vi "RNG.vi"(9 "Minim":dbl, 10 "Maxim":dbl) -> (2 "X val aleatoare":dbl)   [LabVIEW 2024]
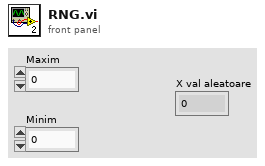
[diagram p1: front panel]
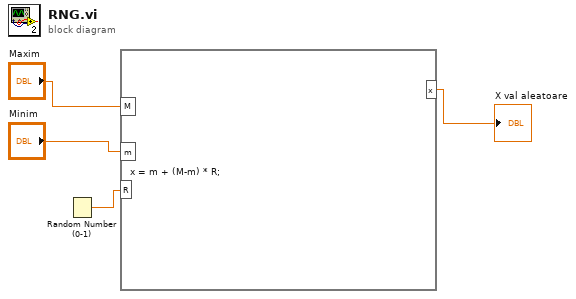
[diagram p0: block diagram]
diagram:
  n1 = Random Number (0-1)() -> (number: 0 to 1=w2:dbl)
  n2 = formula code="x = m + (M-m) * R;"("M"="Maxim", "m"="Minim", "R"=w2) -> ("x"=→"X val aleatoare":dbl)
